vi "GB_DC Bus Test_TS_v2.vi"(8 "error in (no error)":errorcluster, 10 "HMP4040 VISA":refnum<visa-resource-name>, 11 "Control Board VISA":refnum<visa-resource-name>) -> (0 "error out":errorcluster, 3 "Inv_DC":dbl[](array[numeric]))   [LabVIEW 2022 SP3]
uses:
  HMP4040_ChannelControlAutomatic.ctl
  ADCSelector GB.ctl
panel:
  out "INV B (0V)":dbl
  out "INV A (10V)":dbl
  out "INV B (10V)":dbl
  out "INV A (0V)":dbl
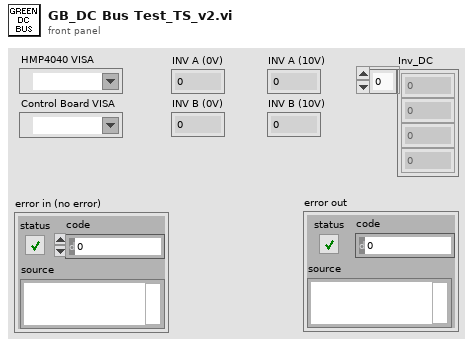
[diagram p1: front panel]
types:
  T1 = typedef "ADCSelector GB.ctl" = enum16{"INVA_ISENSE_U", "INVA_ISENSE_V", "INVA_ISENSE_W", "INVA_UDC", "INVA_TEMP", "HB_ISENSE", "AUX_ISENSE_U", "AUX_ISENSE_V", "AUX_ISENSE_W", "VLINE_AB", "VLINE_BC", "VLINE_CA", "REF_1P5V", "VSENSE_POS_24V", "VSENSE_POS_5V", "VSENSE_NEG_15V", "TEST_POINT", "INVB_ISENSE_U", "INVB_ISENSE_V", "INVB_ISENSE_W", "INVB_UDC", "INVB_TEMP", "HB_TEMP", "AUXA_TEMP", "AUXB_TEMP", "AUXC_TEMP", "VOUT_AB", "VOUT_BC", "VOUT_CA", "REF_2P5V", "VSENSE_POS_15V", "VSENSE_POS_3P3V", "NET_ANALYZER"}
  T2 = typedef "HMP4040_ChannelControlAutomatic.ctl" = enum16{"Off", "Control Power", "HMP2020 Control + DC32V", "HMP2020 Control + DC8V", "HMP4040 Control + DC32V", "HMP4040 Control +DC8V", "HMP4040 Ch2 24V 4A"}
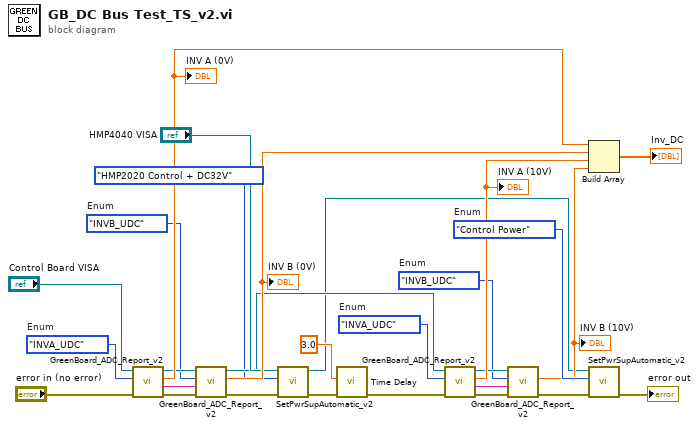
[diagram p0: block diagram]
diagram:
  w3 = ADCSelector_GB."INVB_UDC"  # Enum
  w1 = ADCSelector_GB."INVB_UDC"  # Enum
  w4 = ADCSelector_GB."INVA_UDC"  # Enum
  w2 = ADCSelector_GB."INVA_UDC"  # Enum
  w18 = HMP4040_ChannelControlAutomatic."Control Power"  # Enum
  n1 = call "GreenBoard_ADC_Report_v2.vi"("error in (no error)"="error in (no error)", "Green Board Enum"=w2, "ControlBoard VISA"="Control Board VISA") -> ("error out"=w27:errorcluster, "Message OUT"=w26:string, "Result"=w17:dbl, "VISA Refnum out"=w10:refnum<visa-resource-name>)  [unwired: 5 in]
  "INV A (0V)" <- w17
  n2 = call "GreenBoard_ADC_Report_v2.vi"("error in (no error)"=w27, "Message IN"=w26, "Green Board Enum"=w1, "ControlBoard VISA"=w10) -> ("error out"=w25:errorcluster, "Result"=w16:dbl, "VISA Refnum out"=w9:refnum<visa-resource-name>)  [unwired: 4 in, 1 out]
  "INV B (0V)" <- w16
  n3 = call "SetPwrSupAutomatic_v2.vi"("error in (no error)"=w25, "Enum"=HMP4040_ChannelControlAutomatic."HMP2020 Control + DC32V", "HMP VISA"="HMP4040 VISA") -> ("error out"=w28:errorcluster, "HMP VISA Out"=w5:refnum<visa-resource-name>)  [unwired: 7 in]
  n4 = call "Time Delay"("error in (no error)"=w28, "Delay Time (s)"=3.0) -> ("error out"=w22:errorcluster)  [unwired: 9 in]
  n5 = call "GreenBoard_ADC_Report_v2.vi"("error in (no error)"=w22, "Green Board Enum"=w4, "ControlBoard VISA"=w9) -> ("error out"=w24:errorcluster, "Message OUT"=w23:string, "Result"=w15:dbl, "VISA Refnum out"=w8:refnum<visa-resource-name>)  [unwired: 5 in]
  "INV A (10V)" <- w15
  n6 = call "GreenBoard_ADC_Report_v2.vi"("error in (no error)"=w24, "Message IN"=w23, "Green Board Enum"=w3, "ControlBoard VISA"=w8) -> ("error out"=w20:errorcluster, "Result"=w14:dbl)  [unwired: 4 in, 2 out]
  "INV B (10V)" <- w14
  n7 = Build Array(w17, w16, w15, w14) -> (→"Inv_DC":dbl[])
  n8 = call "SetPwrSupAutomatic_v2.vi"("error in (no error)"=w20, "Enum"=w18, "HMP VISA"=w5) -> ("error out"=→"error out":errorcluster)  [unwired: 7 in, 1 out]
